vi "Stop Bus Controller.vi"(8 "error in":errorcluster, 11 "module handle":u32) -> (0 "error out":errorcluster, 3 "module handle out":u32)   [LabVIEW 2020, in "AIM MIL-STD-1553 Hardware API.lvlib"]
uses:
  AIM MIL-STD-1553 Hardware API.lvlib
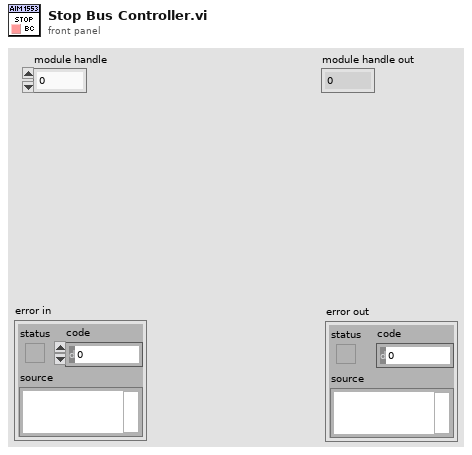
[diagram p1: front panel]
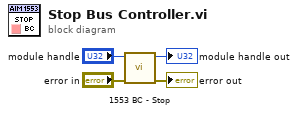
[diagram p0: block diagram]
diagram:
  n1 = call <instrlib>:"1553 BC - Stop.vi"("Error In (none)"="error in", "Module Handle"="module handle") -> ("Error Out"=→"error out":errorcluster, "Module Handle Out"=→"module handle out":u32)  [unwired: 8 in]
